vi "test PID.vi"() -> ()   [LabVIEW 2010]
uses:
  PIDClass.lvclass
panel:
  in  "setpoint 2":dbl=80.0
  in  "stop":bool
  in  "setpoint":dbl=50.0
  out "Waveform Chart":cluster{dbl, dbl}(graph)
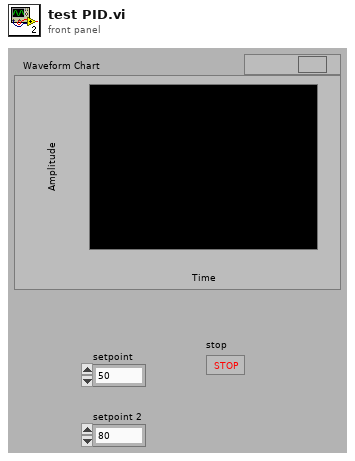
[diagram p1: front panel]
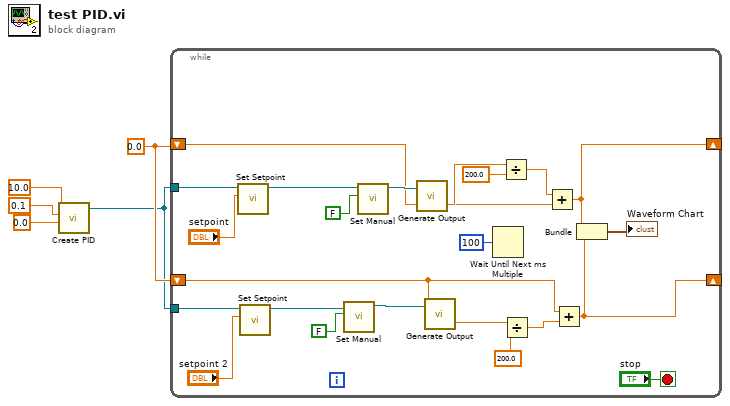
[diagram p0: block diagram]
diagram:
  w5 = 0.0
  n1 = call "Create PID.vi"("D"=0.0, "I"=0.1, "P"=10.0) -> ("PIDClass.lvclass"=w4:refnum<class "PIDClass.lvclass">)  [unwired: 8 out]
  n2 = while {
    tunnel: w4 -> [w6]
    shift-right: [w9] -> _
    shift-left: w5 -> [w24]
    tunnel: w4 -> [w18]
    shift-right: [w10] -> _
    shift-left: w5 -> [w11]
    stop <- "stop" stop-if-true
    n3 = call "Set Setpoint.vi"("setpoint"="setpoint", "PIDClass.lvclass"=w6) -> ("PIDClass.lvclass out"=w7:refnum<class "PIDClass.lvclass">)  [unwired: 9 out]
    n4 = call "Set Setpoint.vi"("setpoint"="setpoint 2", "PIDClass.lvclass"=w18) -> ("PIDClass.lvclass out"=w15:refnum<class "PIDClass.lvclass">)  [unwired: 9 out]
    n5 = call "Set Manual.vi"("Manual"=FALSE, "PIDClass.lvclass"=w15) -> ("PIDClass.lvclass out"=w16:refnum<class "PIDClass.lvclass">)  [unwired: 9 out]
    n6 = call "Set Manual.vi"("Manual"=FALSE, "PIDClass.lvclass"=w7) -> ("PIDClass.lvclass out"=w28:refnum<class "PIDClass.lvclass">)  [unwired: 9 out]
    n7 = call "Generate Output.vi"("Input"=w24, "PIDClass.lvclass"=w28) -> ("Output"=w26:dbl)  [unwired: 1 out]
    n8 = call "Generate Output.vi"("Input"=w11, "PIDClass.lvclass"=w16) -> ("Output"=w13:dbl)  [unwired: 1 out]
    n9 = Wait Until Next ms Multiple(millisecond multiple=u32 100) -> ()  [unwired: 1 out]
    n10 = Divide(x=w26, y=200.0) -> (x/y=w25:dbl)
    n11 = Divide(x=w13, y=200.0) -> (x/y=w12:dbl)
    n12 = Add(x=w25, y=w24) -> (x+y=w9:dbl)
    n13 = Add(x=w11, y=w12) -> (x+y=w10:dbl)
    n14 = Bundle(w9, w10) -> (→"Waveform Chart":cluster{dbl, dbl})  [unwired: 1 out]
  }
